vi "WriteIPaddress.vi"(8 "error in (no error)":errorcluster, 9 "hostname":string="ConnectionInfo.json", 10 "path":path, 11 "ip address":string="ConnectionInfo.json") -> (0 "error out":errorcluster)   [LabVIEW 2017, in "USBDrive.lvlib"]
uses:
  <vilib>/addons/InsightCM/Devices/Shared/Common/USBDrive/USBDrive.lvlib
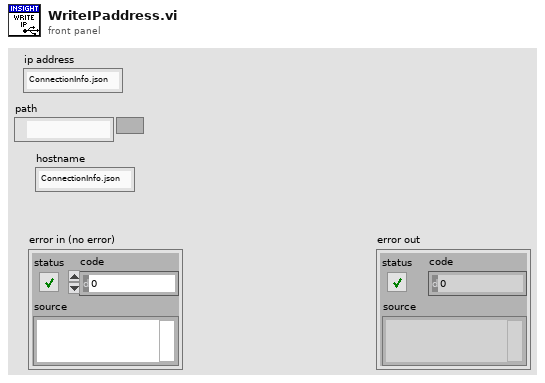
[diagram p1: front panel]
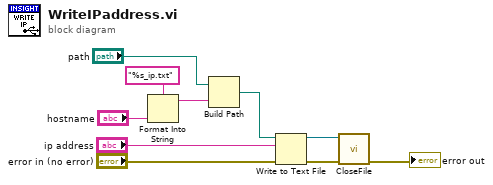
[diagram p0: block diagram]
diagram:
  n1 = Format Into String(format string="%s_ip.txt", "hostname") -> (resulting string=w9:string)  [unwired: 2 in, 1 out]
  n2 = Build Path(base path="path", name or relative path=w9) -> (appended path=w5:path)
  n3 = Write to Text File(file (use dialog)=w5, text="ip address", error in="error in (no error)") -> (refnum out=w3:refnum<file>, error out=w2:errorcluster)  [unwired: 1 in, 1 out]
  n4 = call <vilib>:"CloseFile.vi"("error in (no error)"=w2, "file reference"=w3) -> ("error out"=→"error out":errorcluster)  [unwired: 9 in]
